vi "Log_data_ligne.vi"(10 "test number":string="OCVACIR : ", 11 "test name":string="OCVACIR : ") -> (3 "string out":string)   [LabVIEW 2020]
doc: "Te met en forme les datas pour faire une ligne de log\nex: \"Test# 0 - Test name : ; R = -3.1235 MOhm;\""
uses:
  <userlib>/Alex Log/Log_ligne.ctl
panel:
  in  "data":cluster{"résolution":i16, "resu":dbl, "Type":T1}
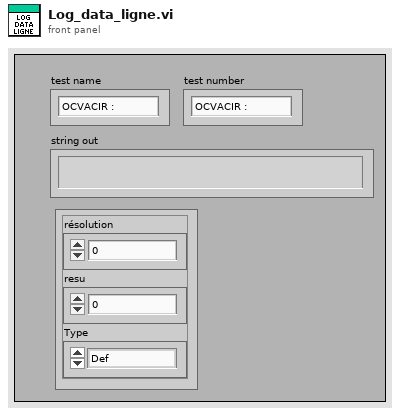
[diagram p1: front panel]
types:
  T1 = typedef "Log_ligne.ctl" = enum16{"Def", "Volt V", "Volt mV", "ohm Ohm", "ohm mOhm", "ohm kOhm", "ohm MOhm"}
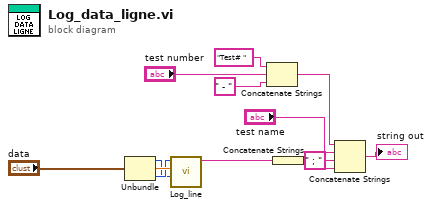
[diagram p0: block diagram]
diagram:
  n1 = Unbundle("data") -> ("résolution"=w2:i16, "resu"=w4:dbl, "Type"=w3:T1)
  n2 = call <userlib>:"Log_line.vi"("résolution"=w2, "resu"=w4, "Type"=w3) -> ("message"=w8:string)  [unwired: 8 in]
  n3 = Concatenate Strings("Test# " ("chaîne"), "test number", " - " ("chaîne")) -> (w9:string)
  n4 = Concatenate Strings(w8) -> (w7:string)
  n5 = Concatenate Strings(w9, "test name", " ; " ("chaîne"), w7) -> (→"string out":string)
